vi "ReadConfigFile.vi"() -> ()   [LabVIEW 2024]
uses:
  <vilib>/Utility/config.llb/Read Key (String).vi
  <vilib>/Utility/config.llb/NI_LVConfig.lvlib
panel:
  out "Menu1":cluster{"Dish Name":string, "Price":dbl}[](array[cluster])
  out "error out":errorcluster
  out "Data":string[][](array[string])
  out "Menu":cluster{"Price":dbl, "Item Name":string}[](array[cluster])
  in  "error in (no error)":errorcluster
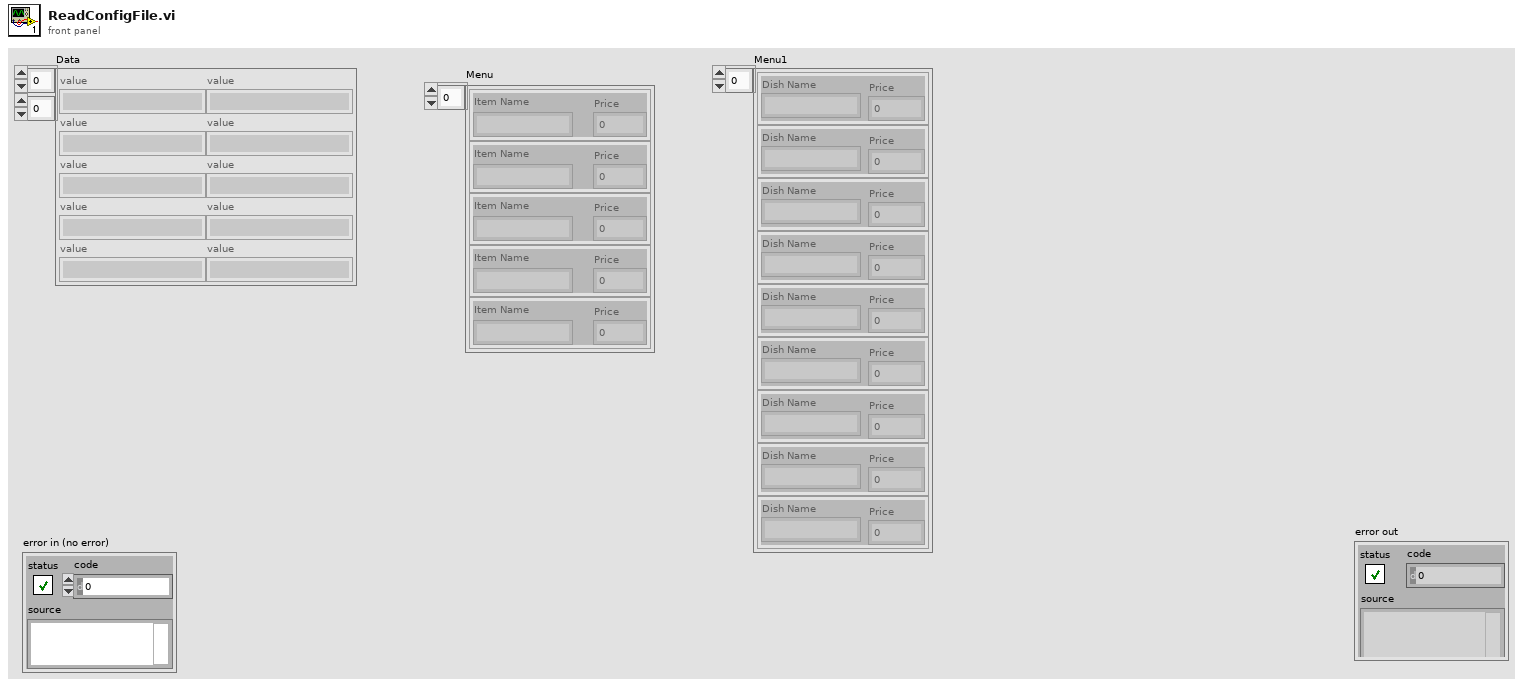
[diagram p1: front panel]
types:
  T1 = typedef "NI_LVConfig.lvlib/Config Data RefNum.ctl" = refnum<k1>
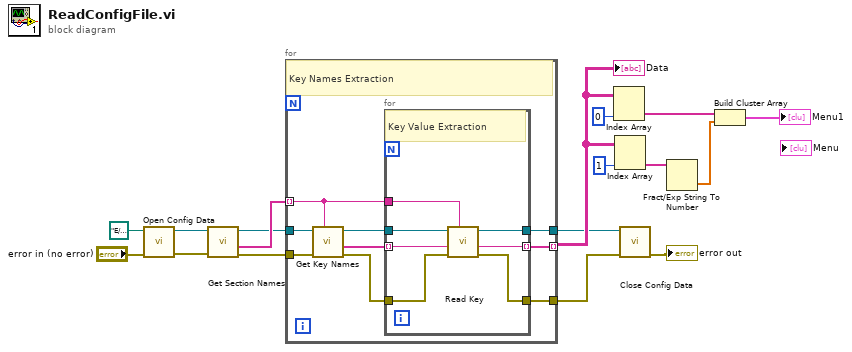
[diagram p0: block diagram]
diagram:
  n1 = call <vilib>:"Open Config Data.vi"("error in (no error)"="error in (no error)", "configuration file path"=path "E:/LabVIEW/Config File/items.ini") -> ("error out"=w14:errorcluster, "refnum"=w15:T1)  [unwired: 7 in, 1 out]
  n2 = call <vilib>:"Get Section Names.vi"("error in (no error)"=w14, "refnum"=w15) -> ("error out"=w11:errorcluster, "section names"=w13:string[], "refnum out"=w12:T1)  [unwired: 7 in]
  n3 = for {
    tunnel: w13 -> [w24] mode=indexing
    tunnel: w12 -> [w26]
    tunnel: w11 -> [w21]
    tunnel: [w20] -> w4
    tunnel: [w19] -> w5
    tunnel: [w18] -> w10 mode=indexing
    # "Key Names Extraction"
    n4 = call <vilib>:"Get Key Names.vi"("section"=w24, "error in (no error)"=w21, "refnum"=w26) -> ("error out"=w22:errorcluster, "key names"=w25:string[], "refnum out"=w23:T1)  [unwired: 5 in, 1 out]
    n5 = for {
      tunnel: w25 -> [w31] mode=indexing
      tunnel: w24 -> [w33]
      tunnel: w23 -> [w32]
      tunnel: [w30] -> w18 mode=indexing
      tunnel: w22 -> [w29]
      tunnel: [w28] -> w20
      tunnel: [w27] -> w19
      # "Key Value Extraction"
      n6 = call-poly <vilib>:"Read Key.vi"("section"=w33, "error in (no error)"=w29, "key"=w31, "refnum"=w32) -> ("error out"=w28:errorcluster, "value"=w30:string, "refnum out"=w27:T1)  [unwired: 4 in, 1 out]
    }
  }
  "Data" <- w10
  n7 = Index Array(array=w10, index (col)=0 ("disabled index (col)")) -> (element=w3:string[])  [unwired: 1 in]
  n8 = Index Array(array=w10, index (col)=1 ("disabled index (col)")) -> (element=w8:string[])  [unwired: 1 in]
  n9 = call <vilib>:"Close Config Data.vi"("error in (no error)"=w4, "refnum"=w5) -> ("error out"=→"error out":errorcluster)  [unwired: 8 in, 1 out]
  n10 = Fract/Exp String To Number(string=w8) -> (number=w2:dbl[])  [unwired: 3 in, 1 out]
  n11 = Build Cluster Array(w3, w2) -> (→"Menu1":cluster{"value":string, "value":dbl}[])
